vi "error_handler.vi"(8 "error in (no error)":errorcluster caption="エラー入力（エラーなし）", 11 "command":T1) -> (0 "error out":errorcluster caption="エラー出力", 3 "error":bool)   [LabVIEW 2015]
uses:
  error_handler_command.ctl
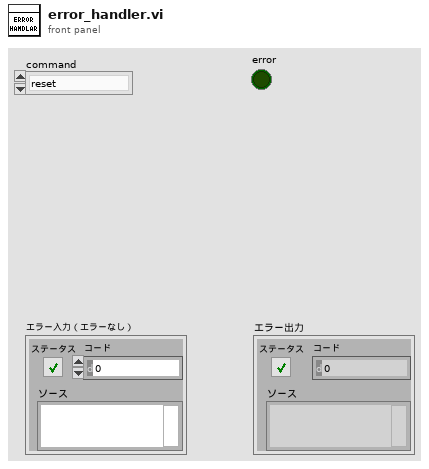
[diagram p1: front panel]
types:
  T1 = typedef "error_handler_command.ctl" = enum16{"reset", "get", "set"}
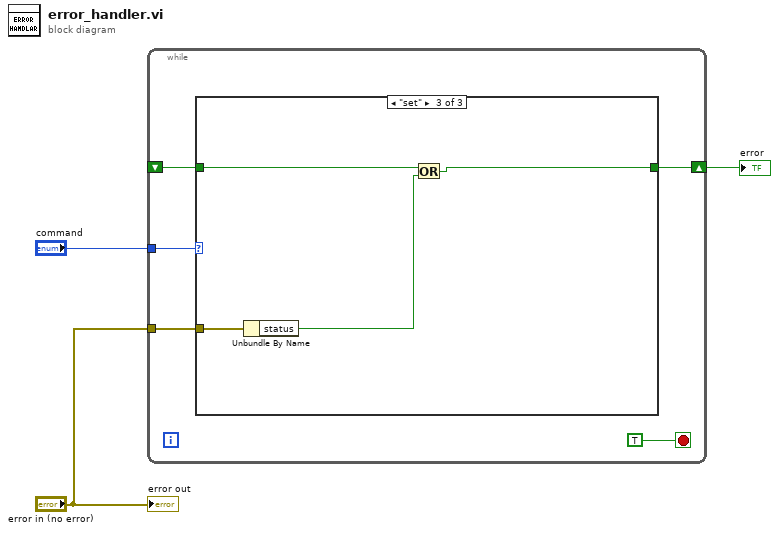
[diagram p0: block diagram]
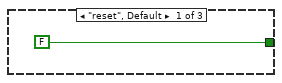
[diagram p2: hidden frame]
diagram:
  n1 = while {
    tunnel: "command" -> [w8]
    shift-right: [w5] -> w1
    shift-left: _ -> [w6]
    tunnel: "error in (no error)" -> [w4]
    stop <- TRUE stop-if-true
    n2 = case shown="\"set\"" w8 {
      tunnel: w6 -> [_ w10 w14]
      tunnel: [FALSE w10 w13] -> w5
      tunnel: w4 -> [_ _ w12]
      frame "reset", Default {
      }
      frame "get" {
      }
      frame "set" {
        n3 = Unbundle By Name(w12) -> ("status"=w11:bool)
        n4 = Or(x=w14, y=w11) -> (x .or. y?=w13:bool)
      }
    }
  }
  "error" <- w1
  "error out" <- "error in (no error)"
